vi "Get_PL_counts.vi"(3 "# of average":i32, 4 "SR400 GPIB Address":string="23") -> (0 "Averaged counts":dbl)   [LabVIEW 2015]
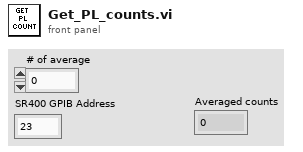
[diagram p1: front panel]
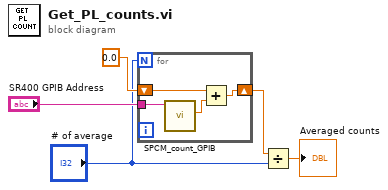
[diagram p0: block diagram]
diagram:
  n1 = for {
    N: "# of average" -> [_]
    shift-right: [w9] -> w3
    shift-left: 0.0 ("Counts") -> [w7]
    tunnel: "SR400 GPIB Address" -> [w6]
    n2 = call "SPCM_count_GPIB.vi"("SR400 GPIB Address"=w6) -> ("Counts"=w8:dbl)  [unwired: 10 in]
    n3 = Add(x=w7, y=w8) -> (x+y=w9:dbl)
  }
  n4 = Divide(x=w3, y="# of average") -> (x/y=→"Averaged counts":dbl)
